vi "LoggingData.vi"(6 "Start time":u32, 8 "error in":errorcluster, 11 "refnum in":refnum<file>) -> (0 "error out":errorcluster, 3 "refnum out":refnum<file>)   [LabVIEW 2017]
uses:
  <vilib>/Rock Robotics/WPI/DriverStation/WPI_DriverStationRobotMode2.ctl
  Framework/Robot Global Data.vi
  Drive/Implementation/Drive Published Globals.vi
  <vilib>/NI_Real-Time Target Support.lvlib
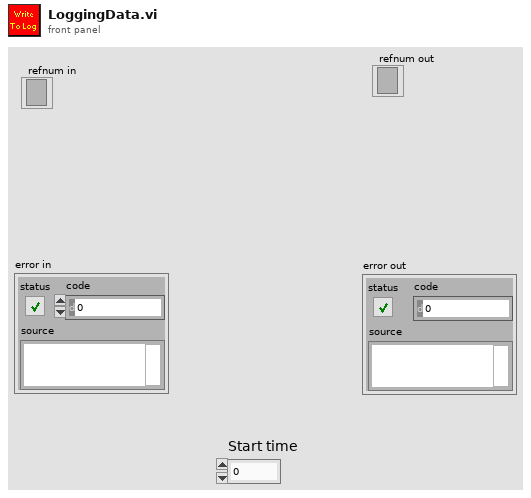
[diagram p1: front panel]
types:
  T1 = typedef "WPI_DriverStationRobotMode2.ctl" = enum16{"Autonomous Disabled", "Autonomous Enabled", "Teleop Disabled", "Teleop Enabled", "Disconnected", "Finish", "Test Disabled", "Test Enabled", "Emergency Stopped"}
  T2 = typedef "Z900_navX_Flags_OpStatusTypeDef.ctl" = u8
  T3 = typedef "Z900_navX_Flags_CalibrationStatusTypeDef.ctl" = u8
  T4 = cluster{"Update Rate Hz":u8, "Accelerometer Full-Scale Range":u8, "Gyro Full-Scale Range":u16, "OP Status":T2, "Calibration Status":T3, "Sensor Status":cluster{"MOVING":bool, "YAW_STABLE":bool, "MAG_DISTURBANCE":bool, "ALTITUDE_VALID":bool, "SEALEVEL_PRESS_SET":bool, "FUSED_HEADING_VALID":bool}, "Self Test Status":cluster{"Gyro Passed":bool, "Accel Passed":bool, "Mag Passed":bool, "Baro Passed":bool, "Complete":bool}}
  T5 = cluster{"MOVING":bool, "YAW_STABLE":bool, "MAG_DISTURBANCE":bool, "ALTITUDE_VALID":bool, "SEALEVEL_PRESS_SET":bool, "FUSED_HEADING_VALID":bool}
  T6 = cluster{"Yaw":dbl, "Roll":dbl, "Pitch":dbl, "Heading":dbl, "Fused Heading":dbl}
  T7 = typedef "NI_Real-Time Target Support.lvlib/RT CPU Load.ctl" = cluster{"Total (%)":dbl, "Time Critical (%)":dbl, "Timed Structures (%)":dbl, "High (%)":dbl, "Above Normal (%)":dbl, "Normal (%)":dbl, "Background (%)":dbl, "Idle (%)":dbl, "ISR (%)":dbl}
  T8 = cluster{"LinearAcceleration X":dbl, "LinearAcceleration Y":dbl, "LinearAcceleration Z":dbl}
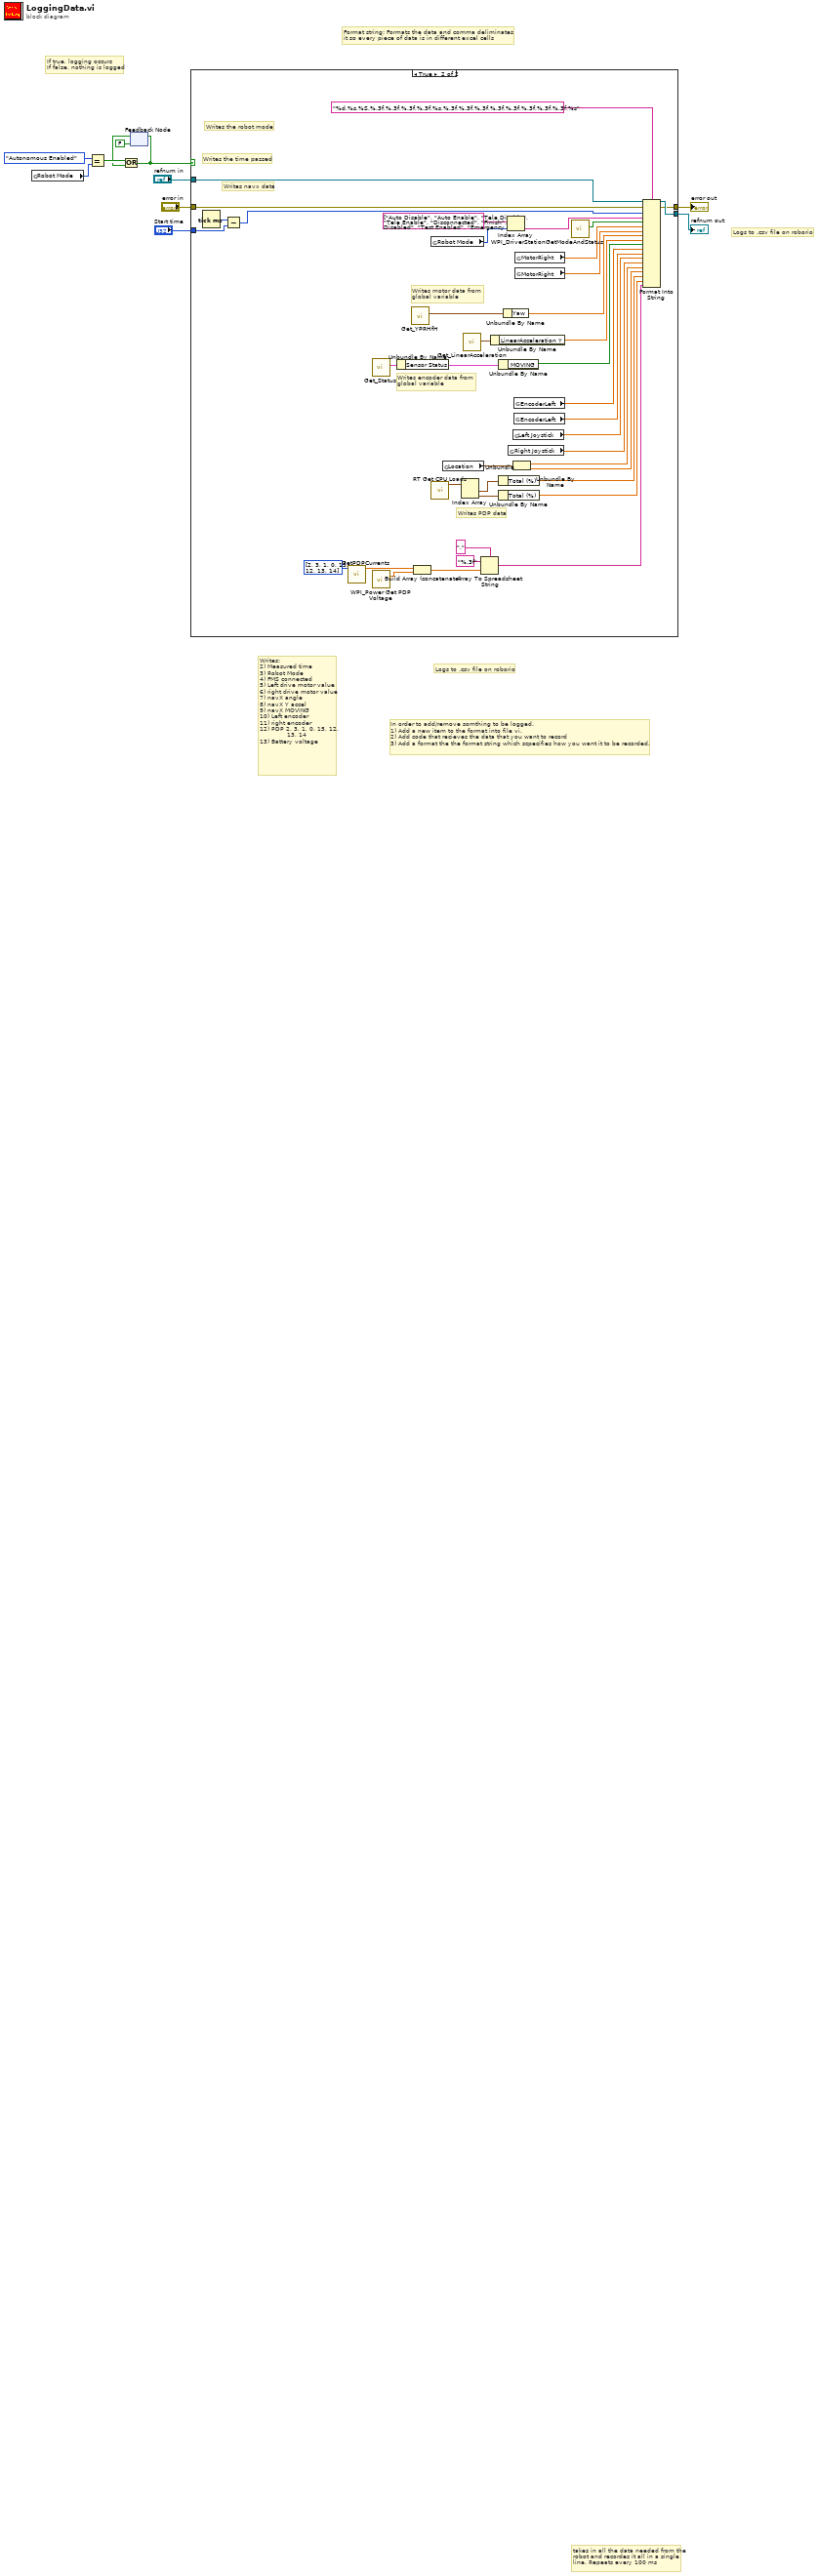
[diagram p0: block diagram]
diagram:
  # "Format string: Formats the data and comma deliminates \nit so every piece of data is in different excel cells"
  # "In order to add/remove somthing to be logged.\n1) Add a new item to the format into file vi.\n2) Add code that recieves the data that you want to record\n3) Add a format the the format string which scpecifies how you want it to be recorded."
  # "Logs to .csv file on roborio"
  # "Writes:\n2) Measured time\n3) Robot Mode\n4) FMS connected\n5) Left drive motor value\n6) right drive motor value\n7) navX angle\n8) navX Y accel\n9) navX MOVING\n10) Left encoder\n11) right encoder\n12) PDP 2, 3, 1, 0, 15, 12,\n              13, 14\n13) Battery voltage"
  # "If true, logging occurs\nIf false, nothing is logged"
  # "takes in all the data needed from the robot and recordes it all in a single line. Repeats every 100 ms"
  # "Logs to .csv file on roborio"
  n1 = global read "Robot Global Data.vi" "Robot Mode"() -> (w6:T1)
  n2 = Equal?(x=WPI_DriverStationRobotMode2."Autonomous Enabled", y=w6) -> (x = y?=w4:bool)
  n3 = feedback #1(FALSE) -> (w3:bool)
  n4 = Or(x=w4, y=w3) -> (x .or. y?=w1:bool)
  n5 = feedback-in #1(w1) -> ()
  n6 = case shown="True" w1 {
    tunnel: "error in" -> [w12 w36]
    tunnel: "refnum in" -> [w13 w38]
    tunnel: [w13 w39] -> w10
    tunnel: [w12 w37] -> w9
    tunnel: "Start time" -> [_ w53]
    frame False {
    }
    frame True {
      # "Writes the time passed"
      # "Writes the robot mode"
      # "Writes motor data from\nglobal variable"
      # "Writes navx data"
      # "Writes encoder data from \nglobal variable"
      # "Writes PDP data"
      n7 = Tick Count (ms)() -> (millisecond timer value=w49:u32)
      n8 = Subtract(x=w49, y=w53) -> (x-y=w35:u32)
      n9 = call "GetPDPCurrents.vi"("Channels"=i32[] [2, 3, 1, 0, 15, 12, 13, 14]) -> ("Currents"=w45:dbl[])  [unwired: 10 in]
      n10 = call <vilib>:"Get_Status.vi"() -> ("Status"=w40:T4)  [unwired: 11 in]
      n11 = call <vilib>:"WPI_Power Get PDP Voltage.vi"() -> ("voltage (V)"=w50:dbl)  [unwired: 14 in, 1 out]
      n12 = Unbundle By Name(w40) -> ("Sensor Status"=w51:T5)
      n13 = call <vilib>:"Get_YPRHfH.vi"() -> ("YRPHfH"=w42:T6)  [unwired: 11 in]
      n14 = Build Array (concatenate)(w45, w50) -> (w46:dbl[])
      n15 = global read "Robot Global Data.vi" "Robot Mode"() -> (w43:T1)
      n16 = call <vilib>:"RT Get CPU Loads.vi"() -> ("CPU loads"=w17:T7[])  [unwired: 10 in, 1 out]
      n17 = global read "Drive Published Globals.vi" "Location"() -> (w22:cluster{dbl, dbl})
      n18 = Index Array(array=w17) -> (element #1=w18:T7, element #2=w19:T7)  [unwired: 2 in]
      n19 = call <vilib>:"Get_LinearAcceleration.vi"() -> ("Linear Acceleration"=w41:T8)  [unwired: 11 in]
      n20 = Array To Spreadsheet String(delimiter (Tab)=",", array=w46, 3:"%.3f" ("format string")) -> (spreadsheet string=w14:string)
      n21 = Unbundle By Name(w41) -> ("LinearAcceleration Y"=w29:dbl)
      n22 = Unbundle By Name(w51) -> ("MOVING"=w28:bool)
      n23 = Unbundle By Name(w18) -> ("Total (%)"=w16:dbl)
      n24 = Unbundle By Name(w19) -> ("Total (%)"=w15:dbl)
      n25 = Unbundle By Name(w42) -> ("Yaw"=w30:dbl)
      n26 = Index Array(array=string[] ["Auto Disable", "Auto Enable", "Tele Disable", "Tele Enable", "Disconnected", "Finish", "Test Disabled", "Test Enabled", "Emergency Stop"], index=w43) -> (element=w34:string)
      n27 = global read "Robot Global Data.vi" "Right Joystick"() -> (w25:dbl)
      n28 = global read "Robot Global Data.vi" "Left Joystick"() -> (w24:dbl)
      n29 = Unbundle(w22) -> (w21:dbl, w20:dbl)
      n30 = global read "Drive Published Globals.vi" "EncoderLeft"() -> (w27:dbl)
      n31 = global read "Drive Published Globals.vi" "EncoderLeft"() -> (w26:dbl)
      n32 = global read "Drive Published Globals.vi" "MotorRight"() -> (w32:dbl)
      n33 = global read "Drive Published Globals.vi" "MotorRight"() -> (w31:dbl)
      n34 = call <vilib>:"WPI_DriverStationGetModeAndStatus.vi"() -> ("FMS Attached"=w33:bool)  [unwired: 10 in, 1 out]
      n35 = Format Into String(format string="%d,%s,%S,%.3f,%.3f,%.3f,%.3f,%s,%.3f,%.3f,%.3f,%.3f,%.3f,%.3f,%.3f,%.3f,%s", initial string=w38, error in=w36, w35, w34, w33, w32, w31, w30, w29, w28, w27, w26, w24, w25, w21, w20, w16, w15, w14) -> (resulting string=w39:refnum<file>, error out=w37:errorcluster)
    }
  }
  "refnum out" <- w10
  "error out" <- w9
